vi "thermometer.vi"() -> ()   [LabVIEW 2018]
doc: "this Vi acquires temp data one value at a time fro, a simulation. It scales the temp and displays it in the thermometer."
panel:
  in  "Numeric":dbl
  out "Thermometer":dbl(slide) scale=0.0..100.0
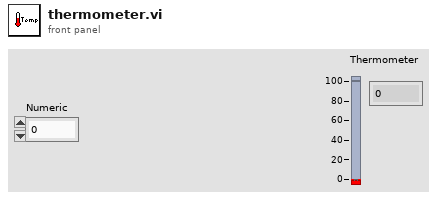
[diagram p1: front panel]
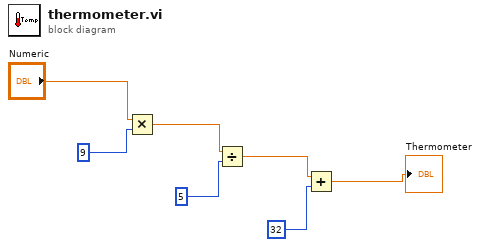
[diagram p0: block diagram]
diagram:
  n1 = Multiply(x="Numeric", y=9) -> (x*y=w5:dbl)
  n2 = Divide(x=w5, y=5) -> (x/y=w3:dbl)
  n3 = Add(x=w3, y=32) -> (x+y=→"Thermometer":dbl)
